vi "ConnectCamera.vi"() -> (0 "error out":errorcluster, 1 "params":variant, 2 "port":u16, 3 "camera":refnum<class "CameraBase.lvclass">)   [LabVIEW 2010]
uses:
  <userlib>/BIAS2/classes/CameraBase/CameraBase.lvclass
  <userlib>/_OpenG.lib/array/array.llb/Search 1D Array (Boolean)__ogtk.vi
  <userlib>/_OpenG.lib/error/error.llb/Filter Error Codes (Array)__ogtk.vi
  <vilib>/addons/h5labview2/file/H5F.lvlib
  <vilib>/addons/h5labview2/attrib/H5A.lvlib
panel:
  in  "offline":bool
  out "h5":path
  in  "cancel":bool
  in  "connect":bool
  in  "cameras":i32(listbox)
  # "Select camera to connect to:"
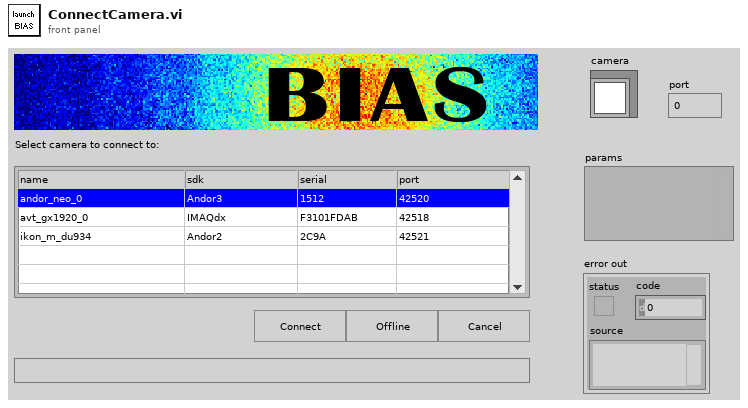
[diagram p1: front panel]
types:
  T1 = typedef "CameraInfo.ctl" = cluster{"name":string, "serial":u64, "interface":string, "make":string, "model":string, "pixel_w":dbl, "pixel_h":dbl}
  T2 = typedef "hid_t.ctl" = i32
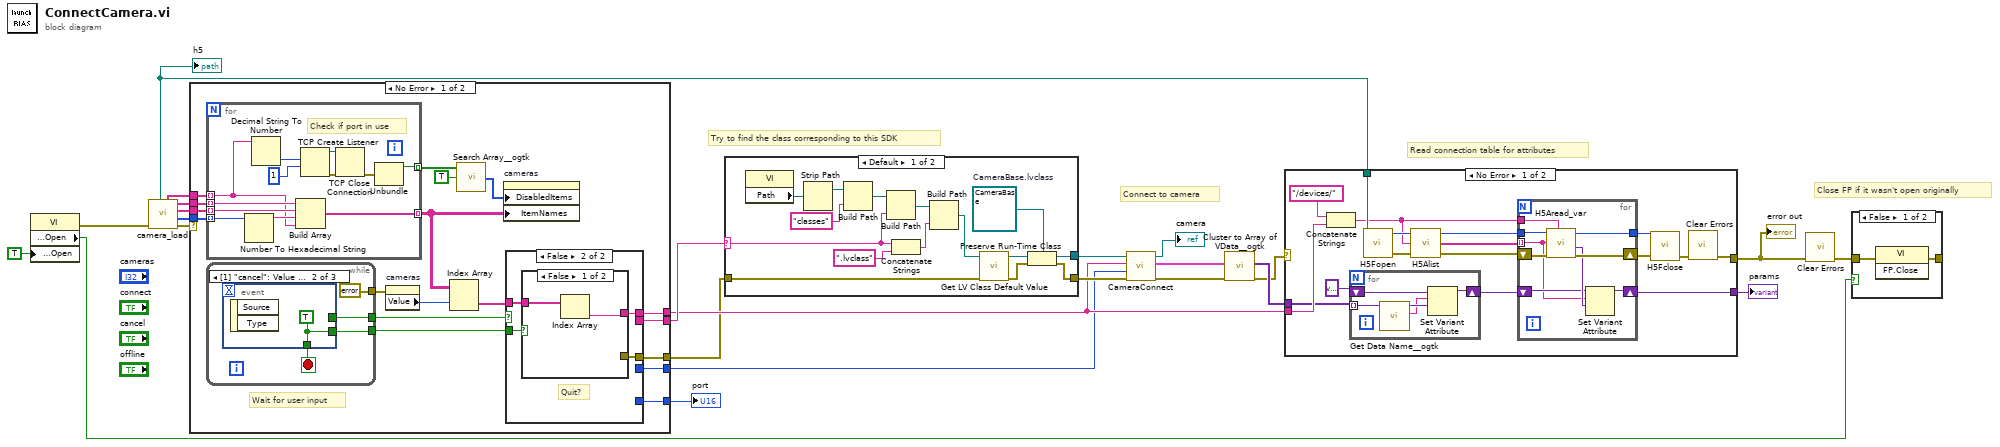
[diagram p0: block diagram]
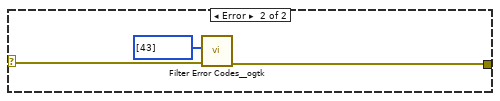
[diagram p4: hidden frame]
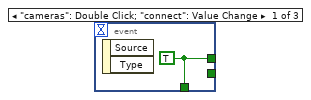
[diagram p5: hidden frame]
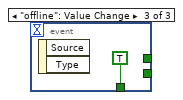
[diagram p6: hidden frame]
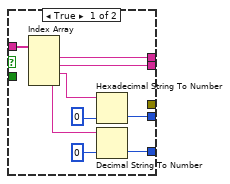
[diagram p7: hidden frame]
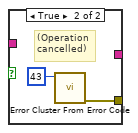
[diagram p8: hidden frame]
diagram:
  # "Close FP if it wasn't open originally"
  # "Connect to camera"
  # "Try to find the class corresponding to this SDK"
  # "Read connection table for attributes"
  n1 = property class="VI"("Front Panel.Open"=TRUE ("Front Panel Window:Open")) -> (error out=w6:errorcluster, "Front Panel.Open"=w2:bool)  [unwired: 2 in, 1 out]
  n2 = call <userlib>:"camera_load.vi"("error in (no error)"=w6) -> ("error out"=w18:errorcluster, "serials"=w24:u64[], "sdks"=w23:string[], "names"=w22:string[], "ports"=w21:string[], "hdf"=w20:path)  [unwired: 3 in]
  "h5" <- w20
  n3 = case shown="No Error" w18 {
    selector: w18 -> [_ w79]
    tunnel: [w42 w79] -> w10
    tunnel: w24 -> [w41 _]
    tunnel: w23 -> [w40 _]
    tunnel: w22 -> [w39 _]
    tunnel: w21 -> [w38 _]
    tunnel: [w37 _] -> w19
    tunnel: [w36 _] -> w12
    tunnel: [w31 _] -> w15
    tunnel: [w30 _] -> w11
    frame No Error {
      # "Wait for user input"
      n4 = for {
        tunnel: w39 -> [w61] mode=indexing
        tunnel: w40 -> [w60] mode=indexing
        tunnel: w41 -> [w59] mode=indexing
        tunnel: [w57] -> w29 mode=indexing
        tunnel: w38 -> [w56] mode=indexing
        tunnel: [w50] -> w35 mode=indexing
        # "Check if port in use"
        n5 = Number To Hexadecimal String(2:w59) -> (0:w58:string)  [unwired: 1 in]
        n6 = Decimal String To Number(string=w56) -> (number=w55:i32)  [unwired: 2 in, 1 out]
        n7 = Build Array(w61, w60, w58, w56) -> (w57:string[])
        n8 = TCP Create Listener(9:1 ("timeout ms (25000)"), 10:w55) -> (0:w53:errorcluster, 3:w52:refnum<k5>)  [unwired: 3 in, 1 out]
        n9 = TCP Close Connection(connection ID=w52, error in (no error)=w53) -> (error out=w51:errorcluster)  [unwired: 1 in, 1 out]
        n10 = Unbundle(w51) -> ("status"=w50:bool)  [unwired: 2 out]
      }
      n11 = while {
        tunnel: [w46] -> w27
        tunnel: [w44] -> w32
        tunnel: [errorcluster {"status"=FALSE, "code"=0, "source"=""} ("error IO")] -> w25
        stop <- w45 stop-if-true
        n12 = event shown="[1] \"cancel\": Value Change;  Panel Close" {
          selector: _ -> [_ _ _]
          dyn-events: _ -> [_ _ _]
          timeout: _ -> [_ _ _]
          tunnel: [w47 _ _] -> w46
          tunnel: [w47 w48 TRUE ("ok")] -> w45
          tunnel: [_ w48 _] -> w44
          event "cameras": Double Click; "connect": Value Change {
            w47 = TRUE ("ok")
            n13 = event-data() -> ()  [unwired: 1 in, 2 out]
          }
          event "cancel": Value Change; Panel Close {
            w48 = TRUE ("ok")
            n14 = event-data() -> ()  [unwired: 1 in, 2 out]
          }
          event "offline": Value Change {
            n15 = event-data() -> ()  [unwired: 1 in, 2 out]
          }
        }
      }
      n16 = property on="cameras" class="MCListbox (strict)"(error in=w25) -> ("Value"=w26:i32)  [unwired: 1 in, 2 out]
      n17 = Index Array(array=w29, index (row)=w26) -> (element=w28:string[])  [unwired: 1 in]
      n18 = call-poly <userlib>:"Search Array__ogtk.vi"("Array"=w35, "Element Data"=TRUE) -> ("Indices of Elements"=w33:i32[])  [unwired: 7 in]
      n19 = property on="cameras" class="MCListbox (strict)"("DisabledItems"=w33, "ItemNames"=w29) -> ()  [unwired: 2 in, 2 out]
      n20 = case shown="False" w27 {
        tunnel: [_ w74] -> w42
        tunnel: [w65 w71] -> w36
        tunnel: [w68 _] -> w37
        tunnel: w32 -> [_ w73]
        tunnel: [w64 _] -> w31
        tunnel: [w63 _] -> w30
        tunnel: w28 -> [w62 w72]
        frame True {
          n21 = Index Array(array=w62) -> (element #1=w65:string, element #2=w64:string, element #3=w67:string, element #4=w69:string)  [unwired: 4 in]
          n22 = Hexadecimal String To Number(string=w67, default (0uL)=u64 0 ("default (0 U32)")) -> (number=w63:u64)  [unwired: 1 in, 1 out]
          n23 = Decimal String To Number(string=w69, default (0L)=u16 0 ("default (0 I32)")) -> (number=w68:u16)  [unwired: 1 in, 1 out]
        }
        frame False {
          # "Quit?"
          n24 = case shown="False" w73 {
            tunnel: [_ w78] -> w74
            tunnel: w72 -> [w76 _]
            tunnel: [w75 _] -> w71
            frame False {
              n25 = Index Array(array=w76) -> (element=w75:string)  [unwired: 1 in]
            }
            frame True {
              # "(Operation\ncancelled)"
              n26 = call <vilib>:"Error Cluster From Error Code.vi"("error code (0)"=43) -> ("error out"=w78:errorcluster)  [unwired: 8 in]
            }
          }
        }
      }
    }
    frame Error {
    }
  }
  "port" <- w19
  n27 = case shown="Default" w15 {
    selector: w15 -> [w88 _]
    tunnel: [w84 _] -> w14
    tunnel: w10 -> [w82 w95]
    tunnel: [w81 w95] -> w13
    frame Default {
      w80 = refnum<class "CameraBase.lvclass"> refnum  # CameraBase.lvclass
      n28 = property on="Property Node" class="VI"() -> ("Path"=w94:path)  [unwired: 2 in, 2 out]
      n29 = Strip Path(path=w94) -> (stripped path=w93:path)  [unwired: 1 out]
      n30 = Build Path(base path=w93, name or relative path="classes") -> (appended path=w91:path)
      n31 = Build Path(base path=w91, name or relative path=w88) -> (appended path=w90:path)
      n32 = Concatenate Strings(w88, ".lvclass" ("string")) -> (w87:string)
      n33 = Build Path(base path=w90, name or relative path=w87) -> (appended path=w89:path)
      n34 = call <vilib>:"Get LV Class Default Value.vi"("error in (no error)"=w82, "class path"=w89) -> ("error out"=w83:errorcluster, "object"=w85:refnum<class>)  [unwired: 8 in]
      n35 = Preserve Run-Time Class(object in=w85, error in=w83, 2:w80) -> (object out=w84:refnum<class "CameraBase.lvclass">, error out=w81:errorcluster)
    }
    frame "" {
      # "Cancelled OR offline"
    }
  }
  n36 = call-dynamic "CameraConnect.vi"("error in (no error)"=w13, "serial"=w11, "name"=w12, "CameraBase in"=w14) -> ("error out"=w1:errorcluster, "CameraInfo"=w9:T1, "CameraBase out"=→"camera":refnum<class "CameraBase.lvclass">)  [unwired: 5 in]
  n37 = call <userlib>:"Cluster to Array of VData__ogtk.vi"("error in (no error)"=w1, "Cluster"=w9) -> ("error out"=w7:errorcluster, "Array of VData"=w8:variant[])  [unwired: 8 in]
  n38 = case shown="No Error" w7 {
    selector: w7 -> [_ w129]
    tunnel: w20 -> [w112 _]
    tunnel: w12 -> [w109 _]
    tunnel: [w97 w128] -> w5
    tunnel: [w96 _] -> w17
    tunnel: w8 -> [w99 _]
    frame No Error {
      n39 = Concatenate Strings("/devices/", w109) -> (w101:string)
      n40 = for {
        tunnel: w99 -> [w124] mode=indexing
        shift-right: [w123] -> w98
        shift-left: variant ("1D Array of Variants") -> [w122]
        n41 = call <userlib>:"Get Data Name__ogtk.vi"("Data"=w124) -> ("Data Name"=w125:string, "Data dup"=w126:variant)  [unwired: 8 in, 1 out]
        n42 = Set Variant Attribute(Variant=w122, name=w125, value=w126) -> (Variant out=w123:variant)  [unwired: 1 in, 2 out]
      }
      n43 = call <vilib>:"H5Fopen.vi"("path"=w112) -> ("error out"=w107:errorcluster, "ref out"=w106:T2)  [unwired: 3 in]
      n44 = call <vilib>:"H5Alist.vi"("error in (no error)"=w107, "object (.)"=w101, "ref in"=w106) -> ("error out"=w103:errorcluster, "attribs"=w102:string[], "ref out"=w105:T2)
      n45 = for {
        tunnel: w105 -> [w120]
        tunnel: [w119] -> w104
        shift-right: [w121] -> w100
        shift-left: w103 -> [w118]
        tunnel: w102 -> [w113] mode=indexing
        tunnel: w101 -> [w117]
        shift-right: [w114] -> w96
        shift-left: w98 -> [w115]
        n46 = call <vilib>:"H5Aread_var.vi"("object name"=w117, "error in (no error)"=w118, "attrib name"=w113, "ref in"=w120) -> ("error out"=w121:errorcluster, "data"=w116:variant, "ref out"=w119:T2)  [unwired: 2 in, 1 out]
        n47 = Set Variant Attribute(Variant=w115, name=w113, value=w116) -> (Variant out=w114:variant)  [unwired: 1 in, 2 out]
      }
      n48 = call <vilib>:"H5Fclose.vi"("error in (no error)"=w100, "ref"=w104) -> ("error out"=w110:errorcluster)  [unwired: 3 in]
      n49 = call <vilib>:"Clear Errors.vi"("error in (no error)"=w110) -> ("error out"=w97:errorcluster)  [unwired: 6 in]
    }
    frame Error {
      n50 = call-poly <userlib>:"Filter Error Codes__ogtk.vi"("Error In"=w129, "Error Codes to Filter"=i32[] [43]) -> ("Error Out"=w128:errorcluster)  [unwired: 7 in, 2 out]
    }
  }
  "params" <- w17
  "error out" <- w5
  n51 = call <vilib>:"Clear Errors.vi"("error in (no error)"=w5) -> ("error out"=w4:errorcluster)  [unwired: 6 in]
  n52 = case shown="False" w2 {
    tunnel: w4 -> [w131 _]
    tunnel: [w130 _] -> _
    frame False {
      n53 = invoke class="VI" method="FP.Close"(error in=w131) -> (error out=w130:errorcluster)  [unwired: 2 in, 2 out]
    }
    frame True {
    }
  }
